vi "Multiple Files Handler.vi"(8 "Error In":errorcluster, 11 "TDMS Log":refnum<class "TDMS Logger.lvclass">) -> (0 "Error Out":errorcluster, 3 "TDMS Log Out":refnum<class "TDMS Logger.lvclass">)   [LabVIEW 2014, in "TDMS Logger.lvlib" / "TDMS Logger.lvclass"]
uses:
  TDMS Logger.lvclass
  TDMS Logger.lvclass/TDMS Logger.ctl
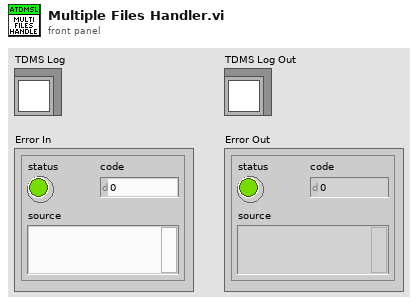
[diagram p1: front panel]
types:
  T1 = typedef "TDMS Logger.lvlib/TDMS Logger.lvclass/Multiple Files Action.ctl" = enum16{"Seperate based on size", "Seperate based on time", "Single file"}
  T2 = enum16{"open", "open or create", "create or replace", "create", "open (read-only)"}
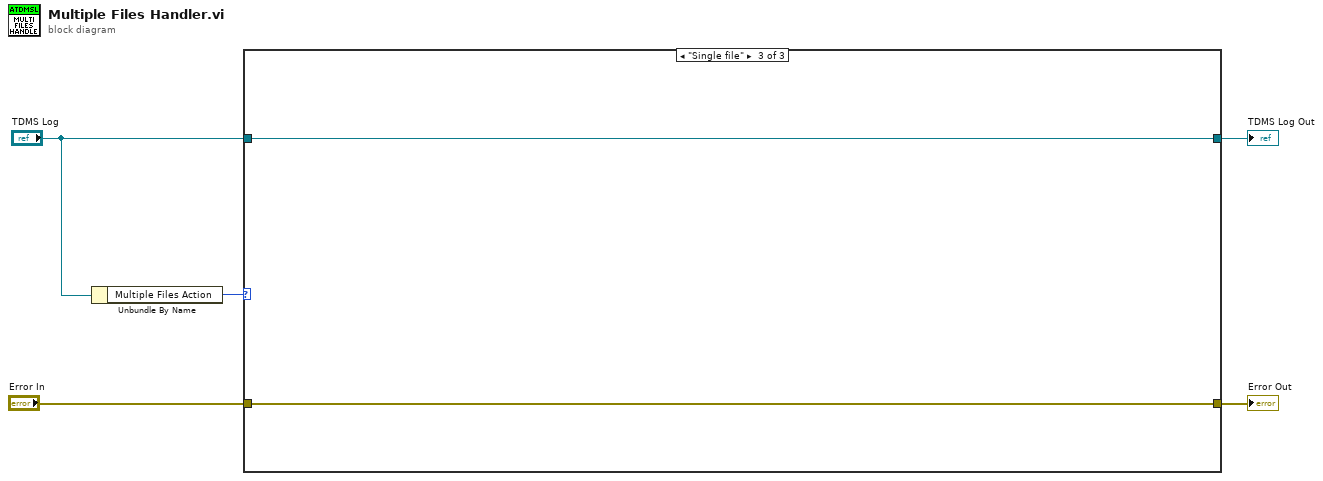
[diagram p0: block diagram]
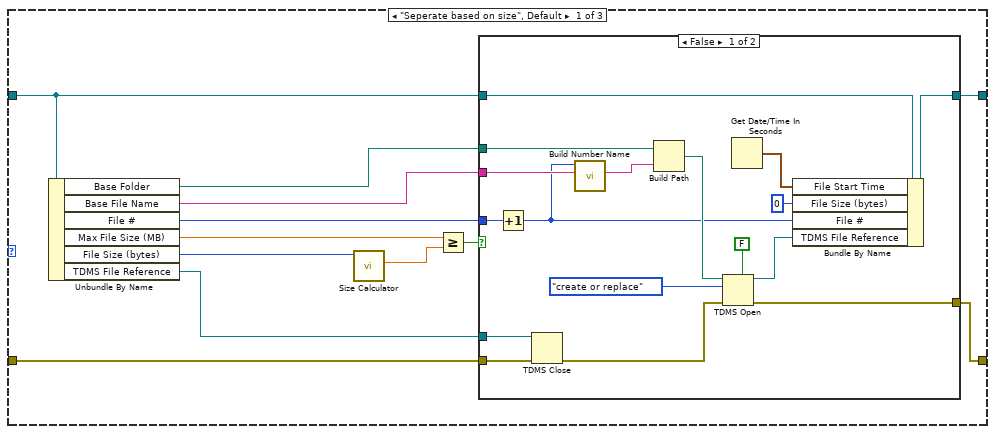
[diagram p2: hidden frame]
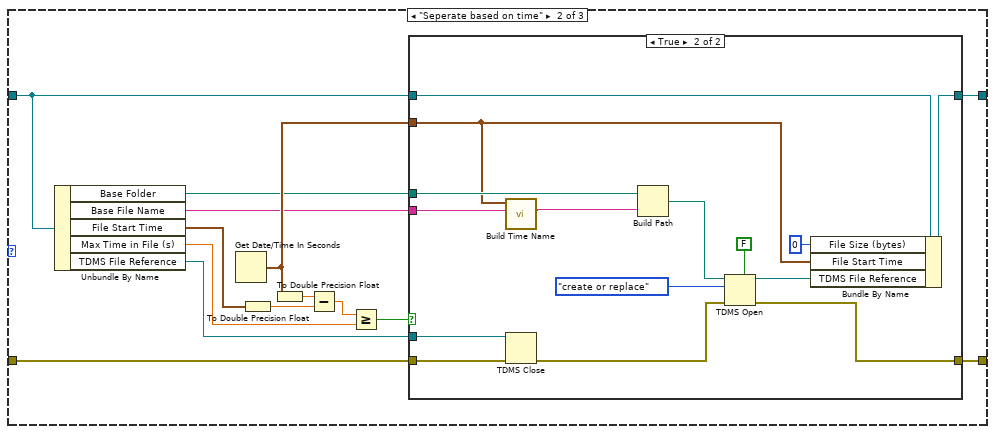
[diagram p4: hidden frame]
diagram:
  n1 = Unbundle By Name("TDMS Log") -> ("Multiple Files Action"=w5:T1)
  n2 = case shown="\"Single file\"" w5 {
    tunnel: [w13 w46 w69] -> w4
    tunnel: "TDMS Log" -> [w14 w47 w69]
    tunnel: "Error In" -> [w6 w45 w68]
    tunnel: [w8 w44 w68] -> w1
    frame "Seperate based on size", Default {
      n3 = Unbundle By Name(w14) -> ("Base Folder"=w9:path, "Base File Name"=w10:string, "File #"=w12:u32, "Max File Size (MB)"=w17:dbl, "File Size (bytes)"=w7:u64, "TDMS File Reference"=w11:refnum<k34>)
      n4 = call "Size Calculator.vi"("Bytes"=w7) -> ("Megabytes"=w16:dbl)  [unwired: 8 in, 2 out]
      n5 = Greater Or Equal?(x=w17, y=w16) -> (x >= y?=w15:bool)
      n6 = case shown="False" w15 {
        tunnel: w14 -> [w34 w36]
        tunnel: [w33 w36] -> w13
        tunnel: w12 -> [w32 _]
        tunnel: w11 -> [w31 _]
        tunnel: w6 -> [w30 w35]
        tunnel: w10 -> [w22 _]
        tunnel: w9 -> [w27 _]
        tunnel: [w24 w35] -> w8
        frame False {
          n7 = Increment(x=w32) -> (x+1=w20:u32)
          n8 = TDMS Close(8:w30, 11:w31) -> (0:w29:errorcluster)  [unwired: 1 out]
          n9 = call "Build Number Name.vi"("Base File Name"=w22, "File #"=w20) -> ("Numbered Name"=w21:string)  [unwired: 9 in]
          n10 = Build Path(base path=w27, name or relative path=w21) -> (appended path=w25:path)
          n11 = TDMS Open(5:FALSE ("create index file? (T)"), 8:w29, 10:T2."create or replace" ("operation (0:open)"), 11:w25) -> (0:w24:errorcluster, 3:w26:refnum<k34>)  [unwired: 3 in]
          n12 = Get Date/Time In Seconds() -> (seconds since 1Jan1904=w18:timestamp)
          n13 = Bundle By Name(cluster=w34, "File Start Time"=w18, "File Size (bytes)"=u64 0, "File #"=w20, "TDMS File Reference"=w26) -> (w33:refnum<class "TDMS Logger.lvclass">)
        }
        frame True {
        }
      }
    }
    frame "Seperate based on time" {
      n14 = Unbundle By Name(w47) -> ("Base Folder"=w40:path, "Base File Name"=w39:string, "File Start Time"=w50:timestamp, "Max Time in File (s)"=w49:dbl, "TDMS File Reference"=w43:refnum<k34>)
      n15 = Get Date/Time In Seconds() -> (seconds since 1Jan1904=w41:timestamp)
      n16 = To Double Precision Float(number=w50) -> (double precision float=w38:dbl)
      n17 = To Double Precision Float(number=w41) -> (double precision float=w37:dbl)
      n18 = Subtract(x=w37, y=w38) -> (x-y=w48:dbl)
      n19 = Greater Or Equal?(x=w48, y=w49) -> (x >= y?=w42:bool)
      n20 = case shown="True" w42 {
        tunnel: w47 -> [w52 w67]
        tunnel: [w52 w66] -> w46
        tunnel: w43 -> [_ w65]
        tunnel: w45 -> [w51 w64]
        tunnel: [w51 w59] -> w44
        tunnel: w41 -> [_ w54]
        tunnel: w40 -> [_ w57]
        tunnel: w39 -> [_ w56]
        frame False {
        }
        frame True {
          n21 = call "Build Time Name.vi"("Base File Name"=w56, "Timestamp"=w54) -> ("Time Name"=w55:string)  [unwired: 9 in]
          n22 = TDMS Close(8:w64, 11:w65) -> (0:w63:errorcluster)  [unwired: 1 out]
          n23 = Build Path(base path=w57, name or relative path=w55) -> (appended path=w60:path)
          n24 = TDMS Open(5:FALSE ("create index file? (T)"), 8:w63, 10:T2."create or replace" ("operation (0:open)"), 11:w60) -> (0:w59:errorcluster, 3:w61:refnum<k34>)  [unwired: 3 in]
          n25 = Bundle By Name(cluster=w67, "File Size (bytes)"=u64 0, "File Start Time"=w54, "TDMS File Reference"=w61) -> (w66:refnum<class "TDMS Logger.lvclass">)
        }
      }
    }
    frame "Single file" {
    }
  }
  "TDMS Log Out" <- w4
  "Error Out" <- w1
